vi "Down Cmd Detect (SubVI).vi"(10 "Read String":string) -> (2 "Down Command":bool)   [LabVIEW 2014]
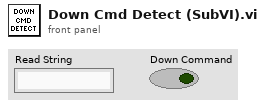
[diagram p1: front panel]
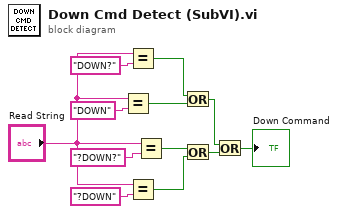
[diagram p0: block diagram]
diagram:
  n1 = Equal?(x="Read String", y="DOWN") -> (x = y?=w9:bool)
  n2 = Equal?(x="Read String", y="DOWN?") -> (x = y?=w8:bool)
  n3 = Equal?(x="Read String", y="?DOWN") -> (x = y?=w6:bool)
  n4 = Equal?(x="Read String", y="?DOWN?") -> (x = y?=w7:bool)
  n5 = Or(x=w8, y=w9) -> (x .or. y?=w11:bool)
  n6 = Or(x=w7, y=w6) -> (x .or. y?=w10:bool)
  n7 = Or(x=w11, y=w10) -> (x .or. y?=→"Down Command":bool)
